vi "meetCriteria.vi"(8 "error in (no error)":errorcluster, 10 "Persons In":refnum<class "Person.lvclass">[](array[class]), 11 "Criteria in":refnum<class "Criteria.lvclass">) -> (0 "error out":errorcluster, 2 "Persons Out":refnum<class "Person.lvclass">[](array[class]), 3 "Criteria out":refnum<class "Criteria.lvclass">)   [LabVIEW 2018, in "Criteria.lvclass"]
uses:
  Criteria.lvclass
  Person Class/Person.lvclass
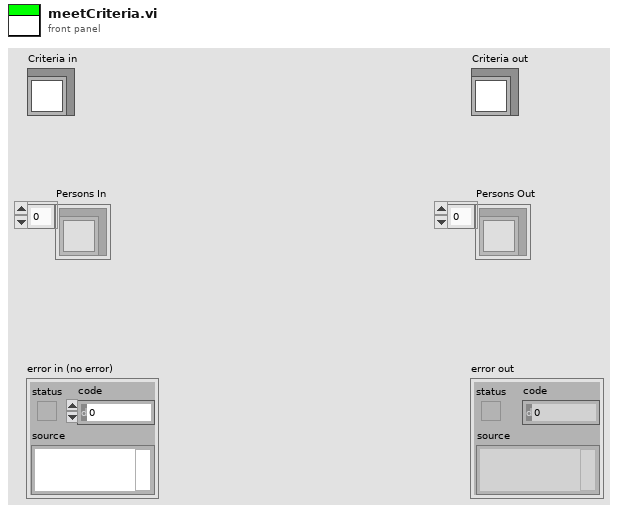
[diagram p1: front panel]
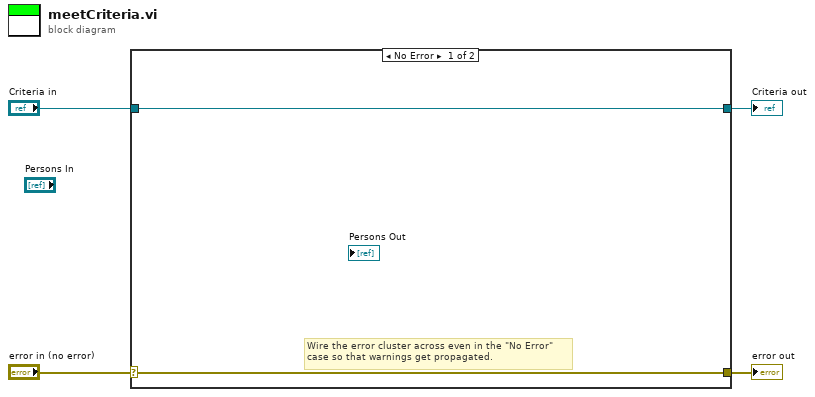
[diagram p0: block diagram]
diagram:
  n1 = case shown="No Error" "error in (no error)" {
    selector: "error in (no error)" -> [w5 w8]
    tunnel: [w5 w8] -> w3
    tunnel: [w6 w7] -> w1
    tunnel: "Criteria in" -> [w6 w7]
    frame No Error {
      # "Wire the error cluster across even in the \"No Error\"\ncase so that warnings get propagated."
    }
    frame Error {
    }
  }
  "error out" <- w3
  "Criteria out" <- w1
